vi "ziGetCurrent.vi"(4 "Opt: DemodVoltage (Vrms)":cdb[](array[numeric]), 5 "PreampCh / Gain(0)":dbl, 7 "ZCtrl / Shunt (0)":dbl, 8 "Error in":errorcluster, 9 "Demodulator (0)":i32, 10 "Mode":T1(ring), 11 "Handle in":T2 {"Handle" format="0x%08x"; "Conn" format="0x%08x"}) -> (0 "Error out":errorcluster, 2 "I (Arms)":cdb[](array[numeric]), 3 "Handle out":T2 {"Handle" format="0x%08x"; "Conn" format="0x%08x"})   [LabVIEW 2009, in "Zurich Instruments LabOne.lvlib"]
doc: "Get the effective current from measured demodulator samples."
uses:
  <instrlib>/Zurich Instruments LabOne/Zurich Instruments LabOne.lvlib
  <instrlib>/Zurich Instruments LabOne/Public/ziTypeHandle.ctl
  <instrlib>/Zurich Instruments LabOne/Public/Utility/Impedance/ziGetCurrentCalcVec.vi
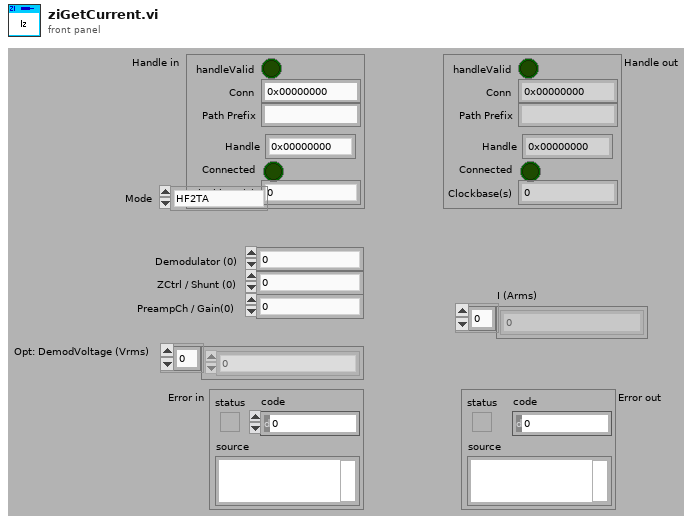
[diagram p1: front panel]
types:
  T1 = enum16{"HF2TA", "HF2CA", "Int. Shunt", "Ext. Shunt"}
  T2 = typedef "Zurich Instruments LabOne.lvlib/ziTypeHandle.ctl" = cluster{"handleValid":bool, "Conn":u64, "Path Prefix":string, "Handle":u64, "Connected":bool, "Clockbase(s)":dbl}
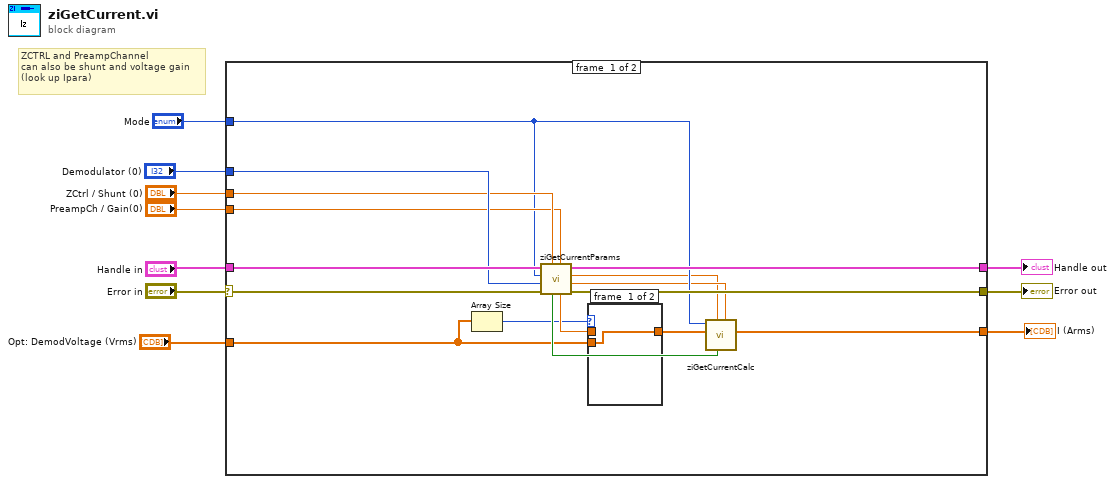
[diagram p0: block diagram]
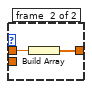
[diagram p2: hidden frame]
diagram:
  # "ZCTRL and PreampChannel\ncan also be shunt and voltage gain\n(look up Ipara)"
  n1 = case shown="No Error" "Error in" {
    selector: "Error in" -> [w25 w30]
    tunnel: "Mode" -> [w17 _]
    tunnel: "ZCtrl / Shunt (0)" -> [w21 _]
    tunnel: "PreampCh / Gain(0)" -> [w20 _]
    tunnel: "Handle in" -> [w23 w31]
    tunnel: [w16 _] -> w2
    tunnel: [w26 w31] -> w7
    tunnel: "Demodulator (0)" -> [w22 _]
    tunnel: [w24 w30] -> w5
    tunnel: "Opt: DemodVoltage (Vrms)" -> [w12 _]
    frame #0 {
      n2 = Array Size(array=w12) -> (size(s)=w11:i32)
      n3 = call <instrlib>:"ziGetCurrentParams.vi"("PreampChannel (0)"=w20, "ZCtrl (0)"=w21, "Error In"=w25, "Demodulator (0)"=w22, "Mode"=w17, "Handle in"=w23) -> ("Error Out"=w24:errorcluster, "VGain"=w15:dbl, "Gain R"=w14:dbl, "Handle Out"=w26:T2, "V (Vrms)"=w18:cdb, "Imp50"=w19:bool)
      n4 = case shown="Default" w11 {
        tunnel: w18 -> [_ w29]
        tunnel: [w27 w28] -> w13
        tunnel: w12 -> [w27 _]
        frame #0 {
        }
        frame #1 {
          n5 = Build Array(w29) -> (w28:cdb[])
        }
      }
      n6 = call-poly <instrlib>:"ziGetCurrentCalc.vi"("VGain"=w15, "Imp50 (F)"=w19, "R"=w14, "DemodVoltage (Vrms)"=w13, "Mode"=w17) -> ("I (Arms)"=w16:cdb[])  [unwired: 6 in]
    }
    frame #1 {
    }
  }
  "Handle out" <- w7
  "Error out" <- w5
  "I (Arms)" <- w2
